vi "Read State.vi"(8 "error in (no error)":errorcluster, 10 "GUI ID":string, 11 "GUI Manager Module in":refnum<class "GUI Manager Module.lvclass">) -> (0 "error out":errorcluster, 2 "GUI State":T1, 3 "GUI Manager Module out":refnum<class "GUI Manager Module.lvclass">)   [LabVIEW 2020, in "VolatusGUI.lvlib" / "GUI Manager Module.lvclass"]
uses:
  GUI Manager Module.lvclass
  GUI State.ctl
  <vilib>/Utility/miscctls.llb/LVRectTypeDef.ctl
  GUI Manager Module.lvclass/GUI Manager Module.ctl
  lv-userprefs/User Prefs/Pref Group/Pref Group.lvclass
  VolatusGUI.lvlib
  lv-vecto/Vecto/Vecto.lvlib
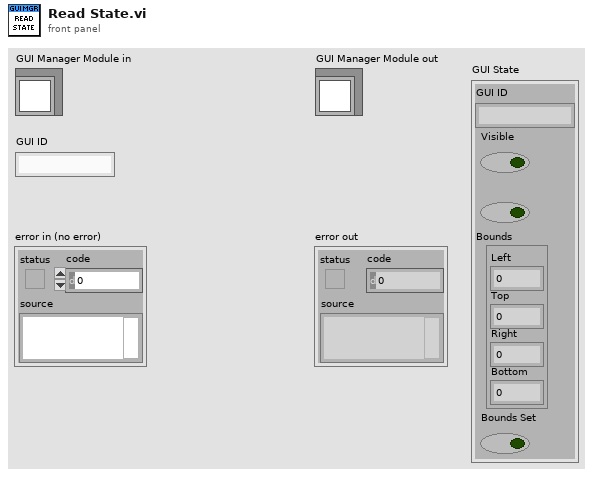
[diagram p1: front panel]
types:
  T1 = typedef "VolatusGUI.lvlib/GUI State.ctl" = cluster{"GUI ID":string, "Visible":bool, "Visibility Set":bool, "Bounds":T2, "Bounds Set":bool}
  T2 = typedef "LVRectTypeDef.ctl" = cluster{"Left":i16, "Top":i16, "Right":i16, "Bottom":i16}
  T3 = cluster{"[0]":i16, "[1]":i16, "[2]":i16, "[3]":i16}
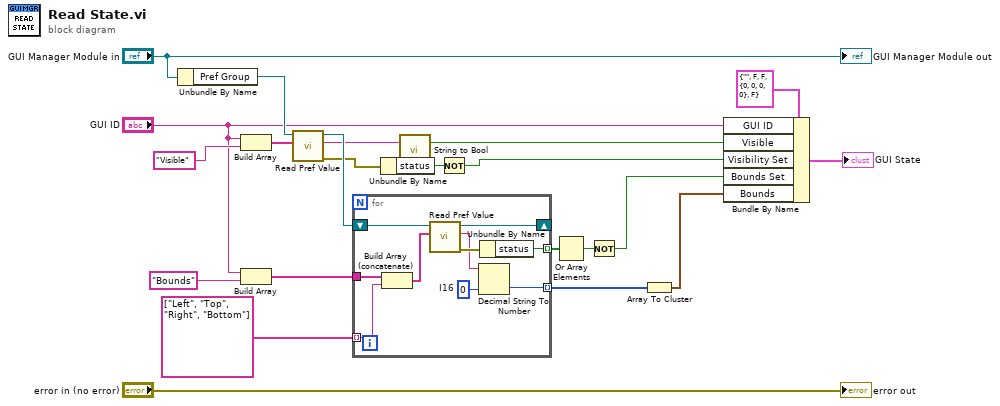
[diagram p0: block diagram]
diagram:
  n1 = Unbundle By Name("GUI Manager Module in") -> ("Pref Group"=w20:refnum<class "Pref Group.lvclass">)
  n2 = Build Array("GUI ID", "Visible" ("GUI ID")) -> (w19:string[])
  n3 = Build Array("GUI ID", "Bounds" ("GUI ID")) -> (w15:string[])
  n4 = call "Read Pref Value.vi"("Pref Hierarchy"=w19, "Pref Group in"=w20) -> ("error out"=w3:errorcluster, "Value"=w12:string, "Pref Group out"=w16:refnum<class "Pref Group.lvclass">)  [unwired: 7 in]
  n5 = for {
    shift-right: [w27] -> _
    shift-left: w16 -> [w31]
    tunnel: w15 -> [w30]
    tunnel: string[] ["Left", "Top", "Right", "Bottom"] -> [w29] mode=indexing
    tunnel: [w24] -> w13 mode=indexing
    tunnel: [w23] -> w6 mode=indexing
    w25 = i16 0  # I16
    n6 = Build Array (concatenate)(w30, w29) -> (w28:string[])
    n7 = call "Read Pref Value.vi"("Pref Hierarchy"=w28, "Pref Group in"=w31) -> ("error out"=w32:errorcluster, "Value"=w26:string, "Pref Group out"=w27:refnum<class "Pref Group.lvclass">)  [unwired: 7 in]
    n8 = Decimal String To Number(string=w26, default (0L)=w25) -> (number=w24:i16)  [unwired: 1 in, 1 out]
    n9 = Unbundle By Name(w32) -> ("status"=w23:bool)
  }
  n10 = Unbundle By Name(w3) -> ("status"=w2:bool)
  n11 = call "String to Bool.vi"("String"=w12) -> ("Bool"=w10:bool)  [unwired: 2 in]
  n12 = Not(x=w2) -> (.not. x?=w1:bool)
  n13 = Or Array Elements(Boolean array=w6) -> (logical OR=w5:bool)
  n14 = Not(x=w5) -> (.not. x?=w4:bool)
  n15 = Array To Cluster(array=w13) -> (cluster=w8:T3)
  n16 = Bundle By Name(cluster=T1 {"GUI ID"="", "Visible"=FALSE, "Visibility Set"=FALSE, "Bounds"={"Left"=0, "Top"=0, "Right"=0, "Bottom"=0}, "Bounds Set"=FALSE} ("GUI State"), "GUI ID"="GUI ID", "Visible"=w10, "Visibility Set"=w1, "Bounds Set"=w4, "Bounds"=w8) -> (→"GUI State":T1)
  "error out" <- "error in (no error)"
  "GUI Manager Module out" <- "GUI Manager Module in"
